vi "SysDef.Search.GUID.vi"(8 "error in (no error)":errorcluster, 10 "GUID":string, 11 "nodeID":u64) -> (0 "error out":errorcluster, 1 "Value out":u64, 3 "nodeID out":u64, 4 "Found?":bool)   [LabVIEW 2015, in "Import - Export CD Config Utility.lvlib"]
uses:
  Import - Export CD Config Utility.lvlib
  <vilib>/NI Veristand/Custom Device Tools/Custom Device Utility Library/NI VeriStand - Search for Item by GUID.vi
  NationalInstruments.VeriStand.SystemDefinitionAPI
  <vilib>/NI Veristand/Custom Device Tools/Custom Device Utility Library/Custom Device Utility Library.lvlib
  NationalInstruments.VeriStand.SystemStorage
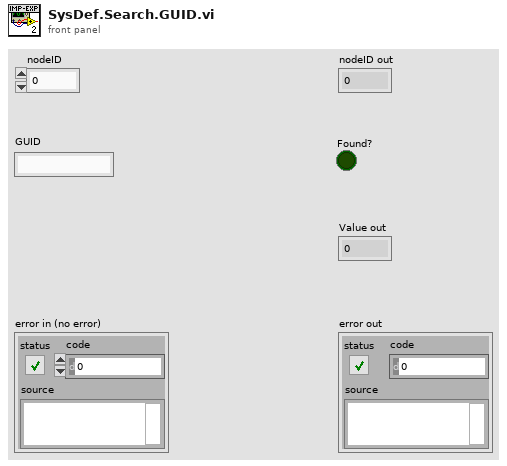
[diagram p1: front panel]
types:
  T1 = typedef "Custom Device API.lvlib/Custom Device Item Ref.ctl" = u64
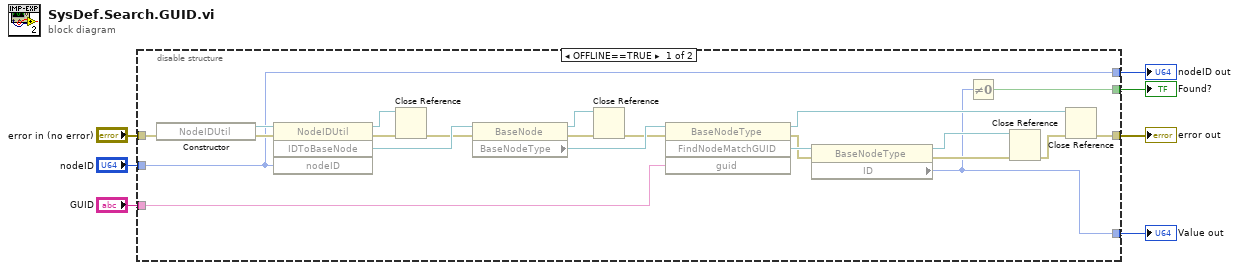
[diagram p0: block diagram]
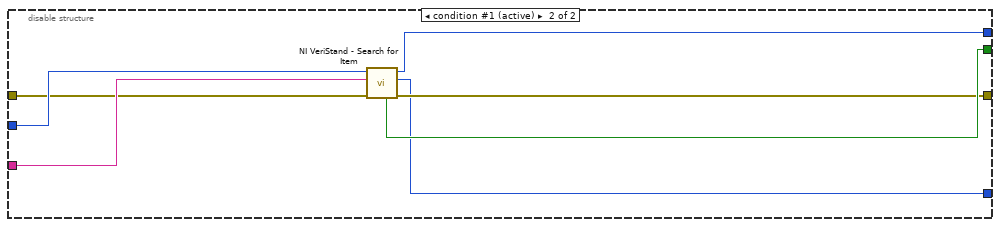
[diagram p2: hidden frame]
diagram:
  n1 = disable-structure shown="OFFLINE==TRUE" {
    disable-tunnel: "error in (no error)" -> [w23 w34]
    disable-tunnel: "nodeID" -> [w19 w35]
    disable-tunnel: [w20 w32] -> w5
    disable-tunnel: "GUID" -> [w17 w36]
    disable-tunnel: [w8 w33] -> w3
    disable-tunnel: [w9 w30] -> w2
    disable-tunnel: [w19 w31] -> w1
    frame condition #0 {
      n2 = constructor class="NodeIDUtil"(error in=w23) -> (reference out=w29:refnum<k24>, error out=w28:errorcluster)  [unwired: 2 in, 1 out]
      n3 = invoke class="NodeIDUtil" method="IDToBaseNode"(reference=w29, error in=w28, "nodeID"=w19) -> (reference out=w24:refnum<k24>, error out=w26:errorcluster, "IDToBaseNode"=w27:refnum<k24>)  [unwired: 1 in, 1 out]
      n4 = Close Reference(reference=w24, error in (no error)=w26) -> (error out=w25:errorcluster)
      n5 = property class="BaseNode"(reference=w27, error in=w25) -> (reference out=w22:refnum<k24>, error out=w21:errorcluster, "BaseNodeType"=w18:refnum<k24>)
      n6 = Close Reference(reference=w22, error in (no error)=w21) -> (error out=w16:errorcluster)
      n7 = invoke class="BaseNodeType" method="FindNodeMatchGUID"(reference=w18, error in=w16, "guid"=w17) -> (reference out=w10:refnum<k24>, error out=w14:errorcluster, "FindNodeMatchGUID"=w15:refnum<k24>)  [unwired: 1 in, 1 out]
      n8 = property class="BaseNodeType"(reference=w15, error in=w14) -> (reference out=w11:refnum<k24>, error out=w13:errorcluster, "ID"=w9:u64)
      n9 = Not Equal To 0?(x=w9) -> (x != 0?=w8:bool)
      n10 = Close Reference(reference=w11, error in (no error)=w13) -> (error out=w12:errorcluster)
      n11 = Close Reference(reference=w10, error in (no error)=w12) -> (error out=w20:errorcluster)
    }
    frame condition #1 (active) {
      n12 = call-poly <vilib>:"NI VeriStand - Search for Item.vi"("error in"=w34, "Item GUID"=w36, "Section Ref in"=w35) -> ("error out"=w32:errorcluster, "Item Ref"=w30:T1, "Section Ref out"=w31:T1, "Found"=w33:bool)  [unwired: 5 in]
    }
  }
  "nodeID out" <- w1
  "error out" <- w5
  "Value out" <- w2
  "Found?" <- w3
